vi "testCAN.vi"() -> ()   [LabVIEW 2015]
uses:
  <vilib>/Utility/Variable/NI_VariableUtilities.lvlib
  Documents/LabVIEW Data/Untitled Project 2/support/Message Queue/Message Cluster.ctl
  <vilib>/Utility/inputDevices.llb/joystickAcquire.vi
  CANFrameControl.ctl
panel:
  out "odeslana predkosc":u16
  out "Waveform Chart 5":cluster{"mean":dbl, "output 3":u16}(graph)
  out "Waveform Chart 2":cluster{"rms value":dbl, "output 2":dbl}(graph)
  out "Numeric 3":dbl
  in  "Boolean":bool
  out "Numeric 2":i32
  in  "stop event":bool
  in  "Tab Control":T1(tab)
  in  "Przód":T2
  out "size(s)":i32[](array[numeric])
  in  "identifier 2":u32 format="%x"
  in  "identifier":u32=1 format="%x"
  in  "stop 2":bool
  out "Ramki CAN":T3[](array[typedef]) {"type" items=["CAN Data", "CAN Remote"]; "identifier" format="%.0x"}
  in  "Adres sbRio":string
  out "Variable4":i64
  out "output 5":u16
  out "output 4":u16
  out "element 2":string
  out "element":string
  out "output 2":u16
  out "output 3":u16
  in  "device index":i32
  in  "Number of Frames to Display":i32=15
  out "Frames":string[][](table)
  in  "stop":bool
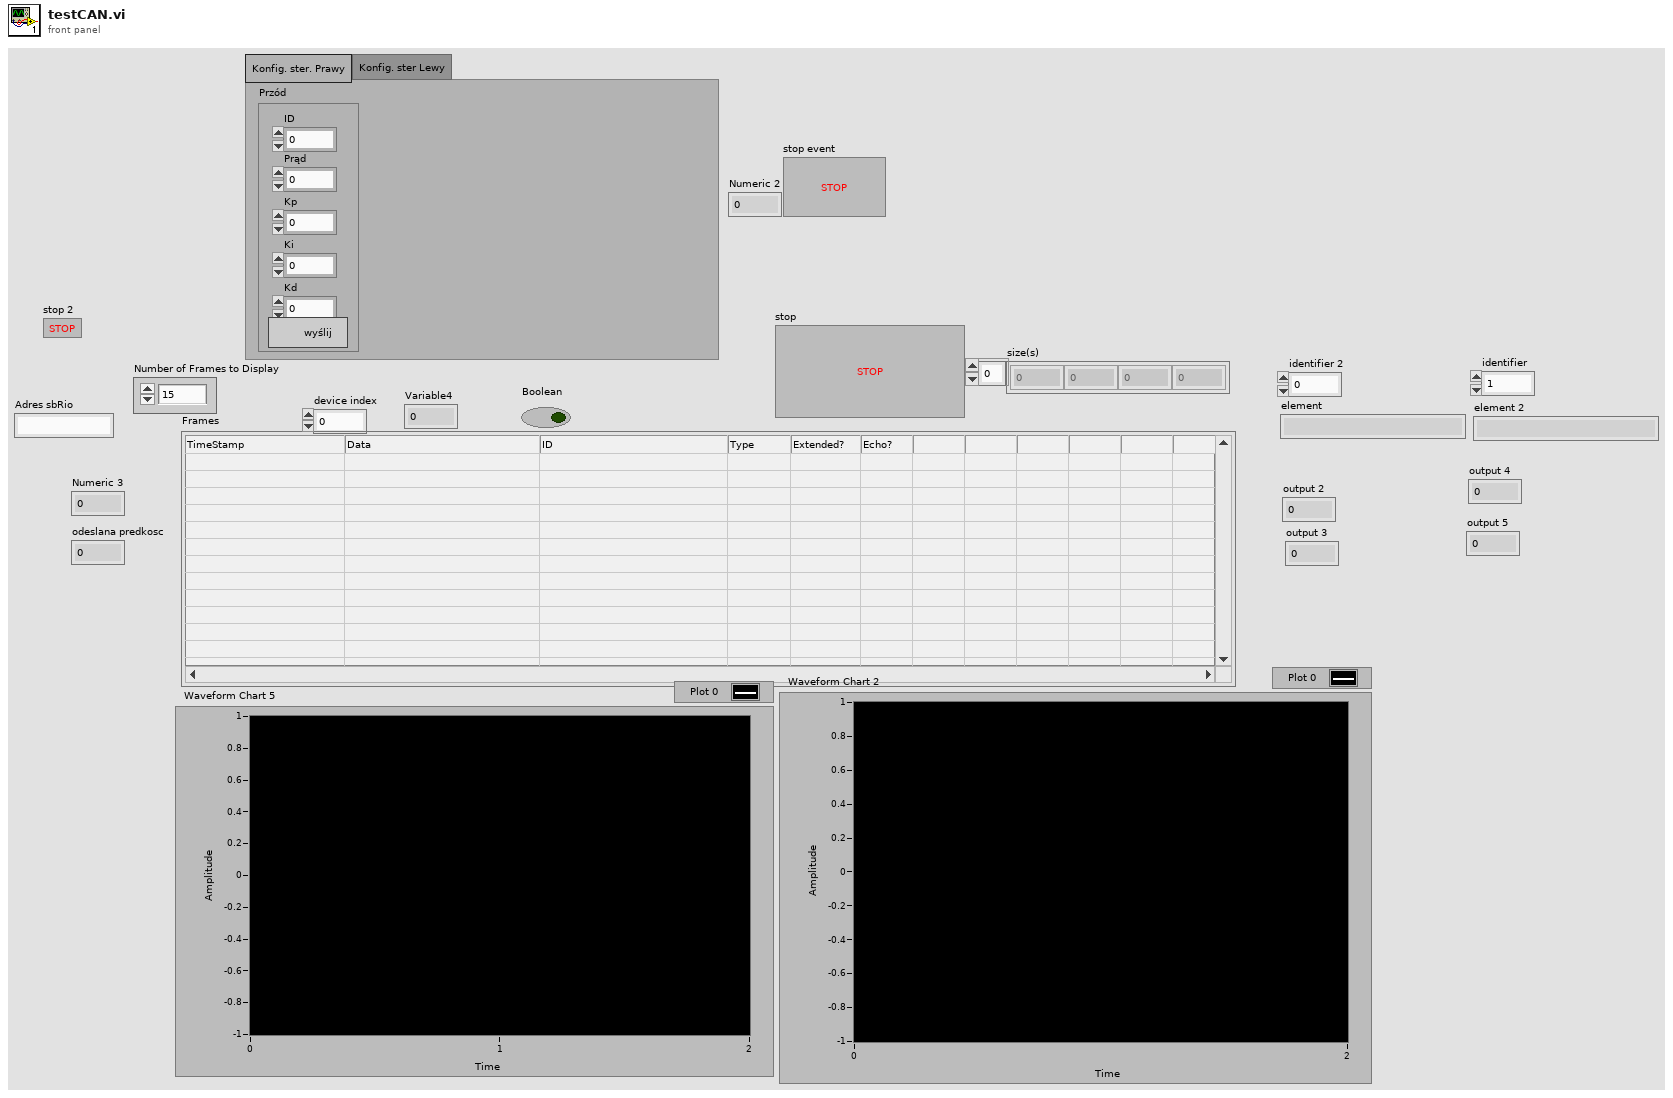
[diagram p1: front panel]
types:
  T1 = enum32{"Konfig. ster. Prawy", "Konfig. ster Lewy"}
  T2 = cluster{"Prąd":u16, "Kp":u16, "Ki":u16, "Kd":u16, "OK Button":bool, "ID":u32}
  T3 = typedef "CANFrameControl.ctl" = cluster{"identifier":u32, "extended?":bool, "type":u8, "payload":u8[]}
  T4 = cluster{"X axis":i32, "Y axis":i32, "Z axis":i32, "X axis rotation":i32, "Y axis rotation":i32, "Z axis rotation":i32, "U axis":i32, "V axis":i32}
  T5 = cluster{"button 1":bool, "button 2":bool, "button 3":bool, "button 4":bool, "button 5":bool, "button 6":bool, "button 7":bool, "button 8":bool, "button 9":bool, "button 10":bool, "button 11":bool, "button 12":bool, "button 13":bool, "button 14":bool, "button 15":bool, "button 16":bool, "button 17":bool, "button 18":bool, "button 19":bool, "button 20":bool, "button 21":bool, "button 22":bool, "button 23":bool, "button 24":bool, "button 25":bool, "button 26":bool, "button 27":bool, "button 28":bool, "button 29":bool, "button 30":bool, "button 31":bool, "button 32":bool}
  T6 = typedef "wyj auto.ctl" = cluster{"AUTO ?":bool, "zadany czas":bool, "Time has Elapsed":bool, "Elapsed Time (s)":dbl, "seconds since 1Jan1904":timestamp}
  T7 = typedef "Message Queue.lvlib/Message Cluster.ctl" = cluster{"Message":string, "Message Data":variant}
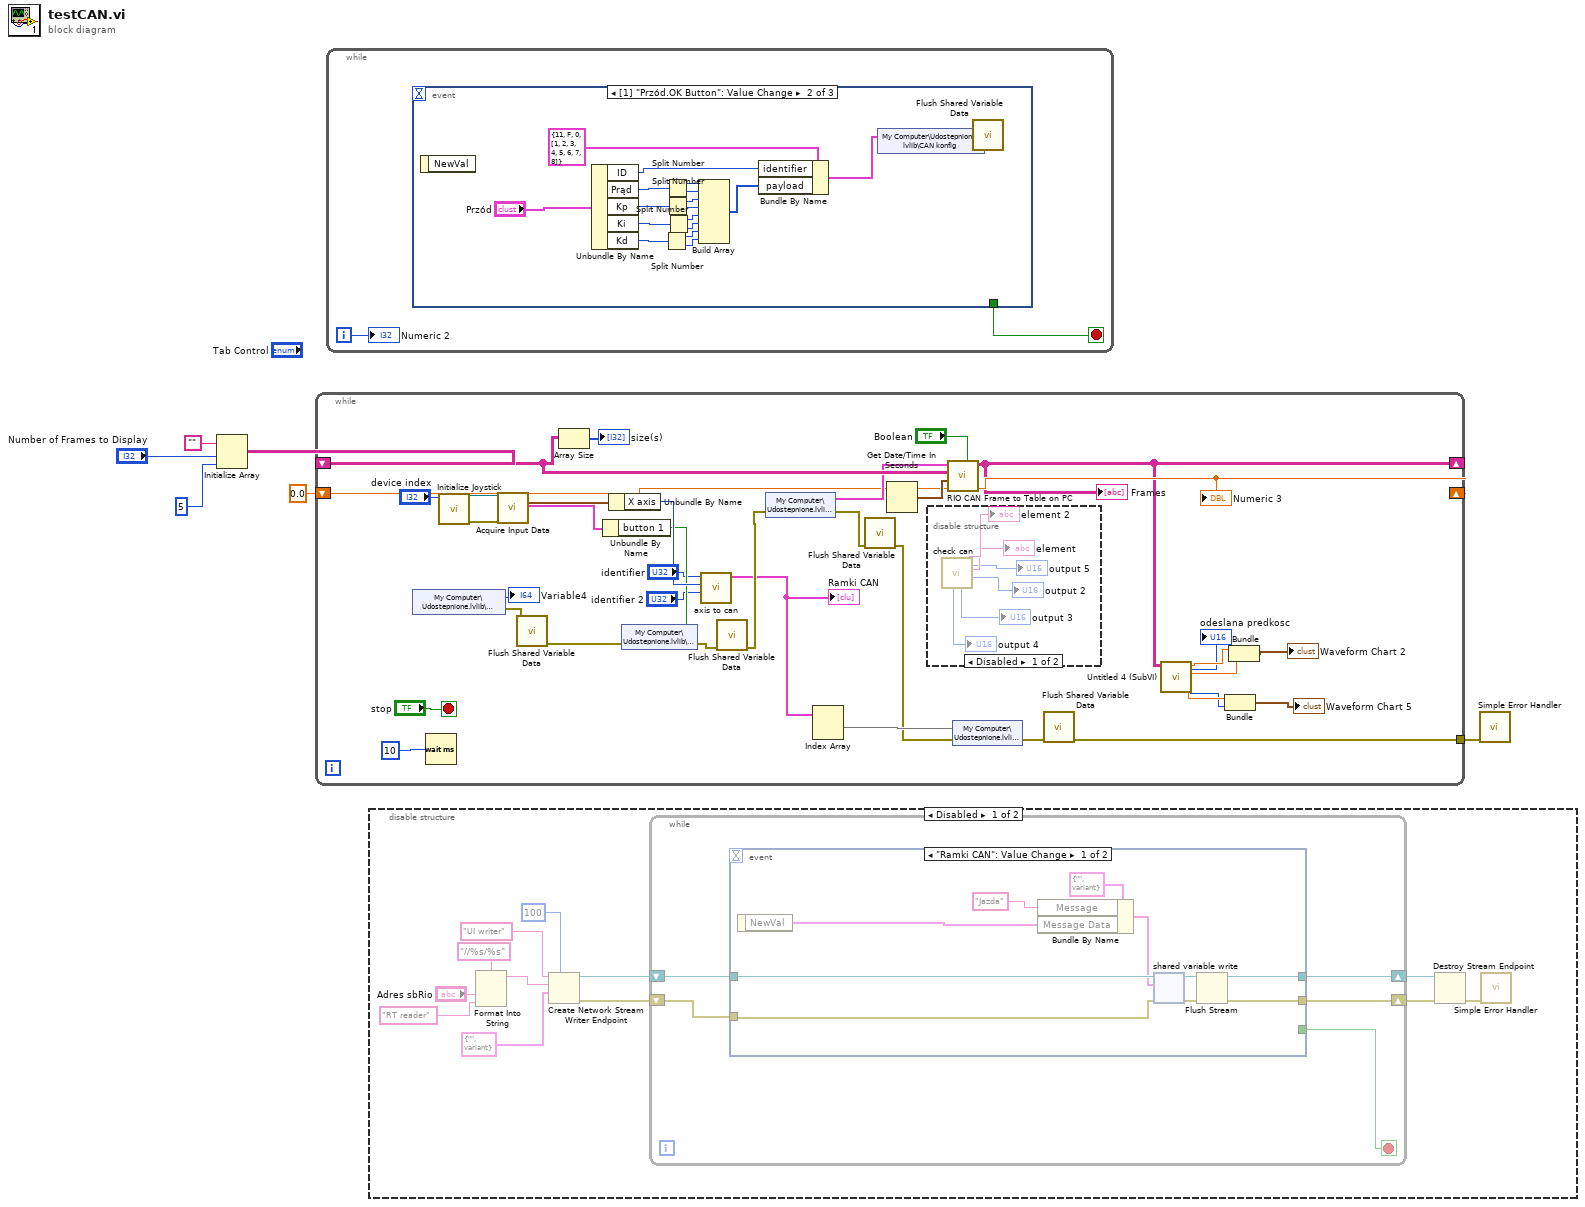
[diagram p0: block diagram]
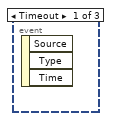
[diagram p2: hidden frame]
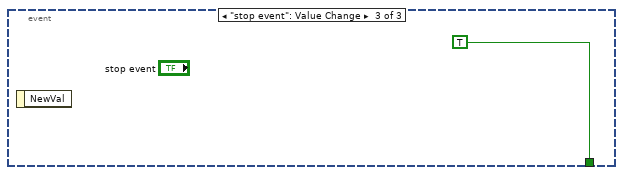
[diagram p3: hidden frame]
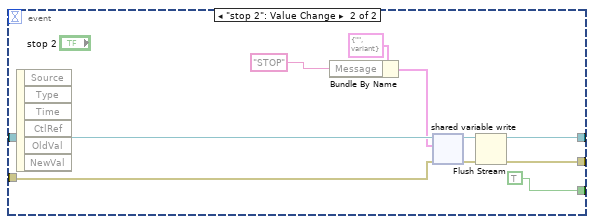
[diagram p4: hidden frame]
diagram:
  n1 = Initialize Array("" ("Empty String Constant"), "Number of Frames to Display", 5 ("dimension size")) -> (w3:string[][])
  n2 = while {
    shift-right: [w7] -> _
    shift-left: w3 -> [w25]
    tunnel: [w18] -> w2
    shift-right: [w17] -> _
    shift-left: 0.0 ("Numeric") -> [w16]
    stop <- "stop" stop-if-true
    n3 = shared-variable "My Computer\\Udostepnione.lvlib\\Variable4"() -> (→"Variable4":i64, error out=w31:errorcluster)  [unwired: 1 in]
    n4 = Wait (ms)(milliseconds to wait=u32 10) -> ()  [unwired: 1 out]
    n5 = call <vilib>:"Initialize Joystick.vi"("device index"="device index") -> ("error out"=w40:errorcluster, "device ID"=w41:refnum<k1>)  [unwired: 9 in]
    n6 = call-poly <vilib>:"Acquire Input Data.vi"("device ID"=w41, "error in (no error)"=w40) -> ("axis info"=w38:T4, "button info"=w37:T5)  [unwired: 13 in, 3 out]
    n7 = call <vilib>:"Flush Shared Variable Data.vi"("error in (no error)"=w31) -> ("error out"=w21:errorcluster)  [unwired: 10 in]
    n8 = Array Size(array=w25) -> (size(s)=→"size(s)":i32[])
    n9 = Unbundle By Name(w37) -> ("button 1"=w34:bool)
    n10 = Unbundle By Name(w38) -> ("X axis"=w36:i32)
    n11 = shared-variable "My Computer\\Udostepnione.lvlib\\status"(w34, error in=w21) -> (error out=w33:errorcluster)
    n12 = call "axis to can.vi"("wej  ID"="identifier 2", "wej wagi"=w36, "ROS in"="identifier") -> ("wyj auto"=w8:T6)  [unwired: 5 in, 3 out]
    "Ramki CAN" <- w8
    n13 = call <vilib>:"Flush Shared Variable Data.vi"("error in (no error)"=w33) -> ("error out"=w20:errorcluster)  [unwired: 10 in]
    n14 = shared-variable "My Computer\\Udostepnione.lvlib\\can2"(error in=w20) -> (w24:cluster{u32, bool, u8, u8[]}, error out=w23:errorcluster)
    n15 = Index Array(array=w8) -> (element #1=w35)  [unwired: 2 in, 1 out]
    n16 = call <vilib>:"Flush Shared Variable Data.vi"("error in (no error)"=w23) -> ("error out"=w19:errorcluster)  [unwired: 10 in]
    n17 = Get Date/Time In Seconds() -> (seconds since 1Jan1904=w26:timestamp)
    n18 = disable-structure shown="Disabled" {
      frame Disabled {
        n19 = call "check can.vi"() -> ("Numeric"=→"output 2":u16, "element"=→"element":string, "element 2"=→"element 2":string, "output 3"=→"output 3":u16, "output 5"=→"output 5":u16, "output 4"=→"output 4":u16)  [unwired: 6 in]
      }
      frame Enabled {
      }
    }
    n20 = call "RIO CAN Frame to Table on PC.vi"("Widok ramek"="Boolean", 8:w16, "timestamp"=w26, "Input CAN Array"=w25, "CAN frame"=w24) -> ("ILE CAN FRAMES"=w17:dbl, "Output CAN Array"=w7:string[][])  [unwired: 2 in, 3 out]
    "Frames" <- w7
    "Numeric 3" <- w17
    n21 = shared-variable "My Computer\\Udostepnione.lvlib\\can1"(w35, error in=w19) -> (error out=w32:errorcluster)
    n22 = call <vilib>:"Flush Shared Variable Data.vi"("error in (no error)"=w32) -> ("error out"=w18:errorcluster)  [unwired: 10 in]
    n23 = call "Untitled 4 (SubVI).vi"("Output Array"=w7) -> ("mean"=w15:dbl, "output 3"=w14:u16, "output 2"=w12:dbl, "rms value"=w13:dbl, "odeslana predkosc"=→"odeslana predkosc":u16)  [unwired: 4 in, 2 out]
    n24 = Bundle("mean"=w15, "output 3"=w14) -> (→"Waveform Chart 5":cluster{"mean":dbl, "output 3":u16})  [unwired: 1 in]
    n25 = Bundle("rms value"=w13, "output 2"=w12) -> (→"Waveform Chart 2":cluster{"rms value":dbl, "output 2":dbl})  [unwired: 1 in]
  }
  n26 = while {
    i -> [w50]
    stop <- w51 stop-if-true
    n27 = event shown="[1] \"Przód.OK Button\": Value Change" {
      selector: _ -> [_ _ _]
      dyn-events: _ -> [_ _ _]
      timeout: _ -> [_ _ _]
      tunnel: [_ _ TRUE] -> w51
      event Timeout {
        n28 = event-data() -> ()  [unwired: 1 in, 3 out]
      }
      event "Przód.OK Button": Value Change {
        n29 = event-data() -> ()  [unwired: 1 in, 1 out]
        n30 = Unbundle By Name("Przód") -> ("ID"=w55:u32, "Prąd"=w59:u16, "Kp"=w58:u16, "Ki"=w57:u16, "Kd"=w56:u16)
        n31 = Split Number(x=w56) -> (hi(x)=w61:u8, lo(x)=w60:u8)
        n32 = Split Number(x=w59) -> (hi(x)=w67:u8, lo(x)=w66:u8)
        n33 = Split Number(x=w58) -> (hi(x)=w65:u8, lo(x)=w64:u8)
        n34 = Split Number(x=w57) -> (hi(x)=w63:u8, lo(x)=w62:u8)
        n35 = Build Array(w67, w66, w65, w64, w63, w62, w61, w60) -> (w68:u8[])
        n36 = Bundle By Name(cluster=T3 {"identifier"=11, "extended?"=FALSE, "type"=0, "payload"=[1, 2, 3, 4, 5, 6, 7, 8]} ("CAN frame 3"), "identifier"=w55, "payload"=w68) -> (w52:T3)
        n37 = shared-variable "My Computer\\Udostepnione.lvlib\\CAN konfig"(w52) -> (error out=w54:errorcluster)  [unwired: 1 in]
        n38 = call <vilib>:"Flush Shared Variable Data.vi"("error in (no error)"=w54) -> ()  [unwired: 10 in, 1 out]
      }
      event "stop event": Value Change {
        n39 = event-data() -> ()  [unwired: 1 in, 1 out]
      }
    }
    "Numeric 2" <- w50
  }
  n40 = disable-structure shown="Disabled" {
    frame Disabled {
      n41 = Format Into String(format string="//%s/%s", "Adres sbRio", "RT reader" ("writer name")) -> (resulting string=w80:string)  [unwired: 2 in, 1 out]
      n42 = Create Network Stream Writer Endpoint(7:100 ("writer buffer size"), 9:T7 {"Message"="", "Message Data"=variant} ("Message Cluster"), 10:w80, 11:"UI writer" ("writer name")) -> (0:w76:errorcluster, 3:w77:refnum<k21>)  [unwired: 3 in]
      n43 = while {
        shift-right: [w87] -> w74
        shift-left: w77 -> [w88]
        shift-right: [w86] -> w73
        shift-left: w76 -> [w85]
        i -> [w83]
        stop <- w84 stop-if-true
        n44 = event shown="[0] \"Ramki CAN\": Value Change" {
          selector: _ -> [_ _]
          dyn-events: _ -> [_ _]
          timeout: _ -> [_ _]
          tunnel: w88 -> [w95 w105]
          tunnel: [w92 w102] -> w87
          tunnel: [w91 w101] -> w86
          tunnel: w85 -> [w90 w100]
          tunnel: [_ TRUE] -> w84
          event "Ramki CAN": Value Change {
            n45 = event-data() -> ("NewVal"=w89:T3[])  [unwired: 1 in]
            n46 = Bundle By Name(cluster=T7 {"Message"="", "Message Data"=variant} ("Message Cluster"), "Message"="Jazda", "Message Data"=w89) -> (w94:T7)
            n47 = shared-variable-write(w95, w90, w94) -> (w97:refnum<k21>, w98:errorcluster)  [unwired: 1 in, 1 out]
            n48 = Flush Stream(8:w98, 11:w97) -> (0:w91:errorcluster, 3:w92:refnum<k21>)  [unwired: 2 in, 1 out]
          }
          event "stop 2": Value Change {
            n49 = event-data() -> ()  [unwired: 1 in, 6 out]
            n50 = Bundle By Name(cluster=T7 {"Message"="", "Message Data"=variant} ("Message Cluster"), "Message"="STOP") -> (w104:T7)
            n51 = shared-variable-write(w105, w100, w104) -> (w107:refnum<k21>, w108:errorcluster)  [unwired: 1 in, 1 out]
            n52 = Flush Stream(8:w108, 11:w107) -> (0:w101:errorcluster, 3:w102:refnum<k21>)  [unwired: 2 in, 1 out]
          }
        }
      }
      n53 = Destroy Stream Endpoint(8:w73, 11:w74) -> (0:w75:errorcluster)
      n54 = call <vilib>:"Simple Error Handler.vi"("error in (no error)"=w75) -> ()  [unwired: 4 in, 5 out]
    }
    frame Enabled {
    }
  }
  n55 = call <vilib>:"Simple Error Handler.vi"("error in (no error)"=w2) -> ()  [unwired: 4 in, 5 out]
